vi "Maxi Gauge-Driver Core.vi"(0 "VISA-Ressource in":refnum<visa-resource-name>, 1 "Write/Read":bool, 5 "Node address":i8=-1 min=-1 max=31 step=1, 7 "Command":string, 11 "Fehler (Eingang)":errorcluster, 12 "Timeout [ms]":u32=600 min=1 max=20000 step=1, 13 "Retry (3)":i32=3 min=1 max=20000 step=1) -> (4 "VISA-Ressource out":refnum<visa-resource-name>, 8 "String Out":string, 15 "Fehler (Ausgang)":errorcluster)   [LabVIEW 2018, in "Maxi Gauge.lvlib"]
uses:
  Maxi Gauge.lvlib
panel:
  in  "ENQ [\\05]":string="\u0005"
  in  "NAK [\\15]":string="\u0015"
  in  "ACK [\\06]":string="\u0006"
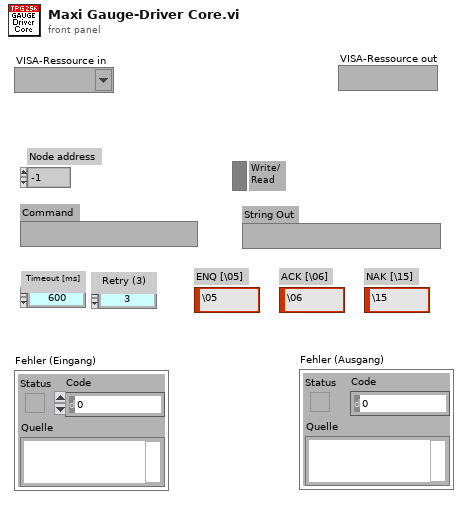
[diagram p1: front panel]
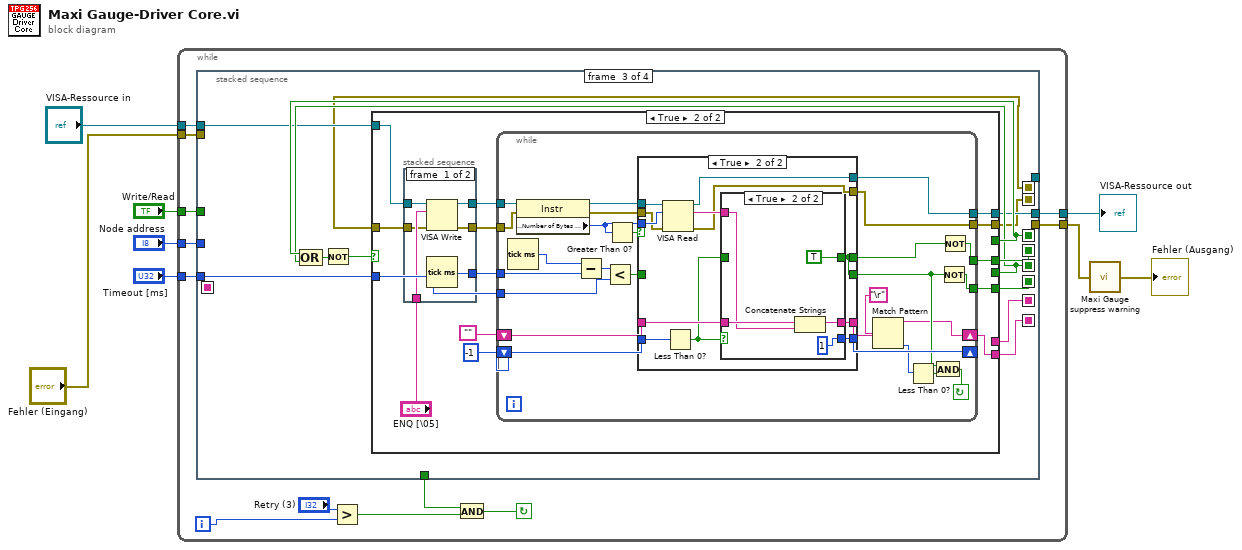
[diagram p0: block diagram]
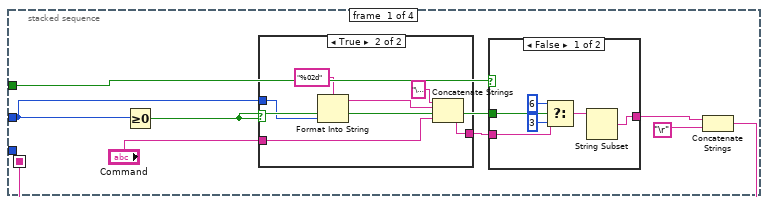
[diagram p2: hidden frame]
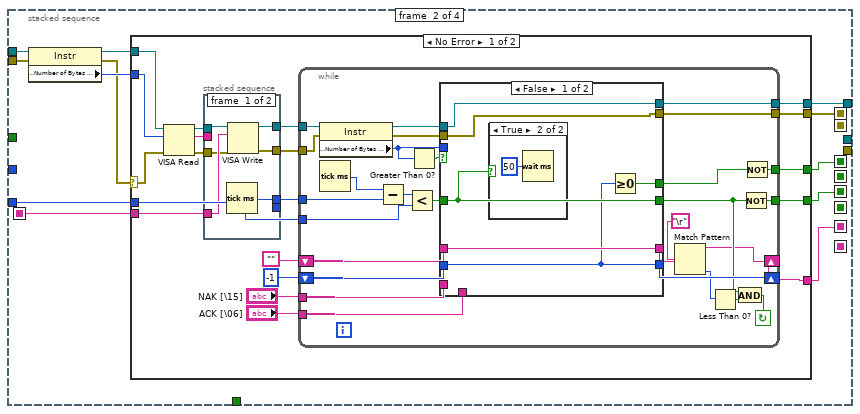
[diagram p5: hidden frame]
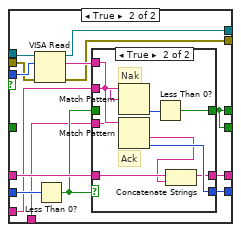
[diagram p7: hidden frame]
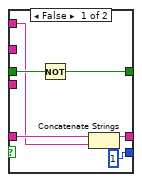
[diagram p8: hidden frame]
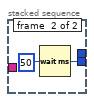
[diagram p9: hidden frame]
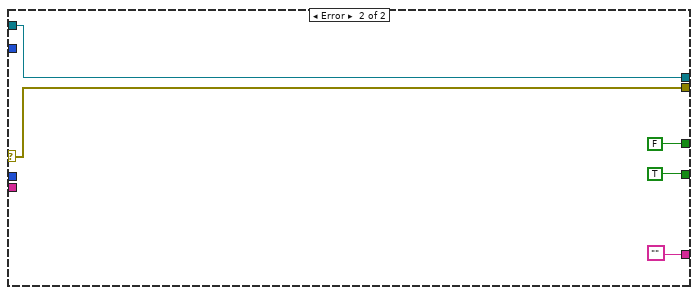
[diagram p10: hidden frame]
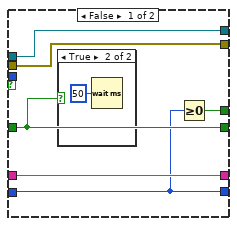
[diagram p12: hidden frame]
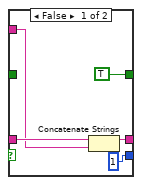
[diagram p14: hidden frame]
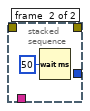
[diagram p15: hidden frame]
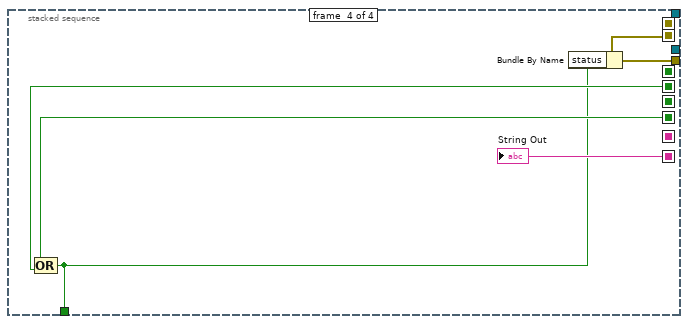
[diagram p16: hidden frame]
diagram:
  n1 = while {
    tunnel: "Node address" -> [w13]
    tunnel: "Write/Read" -> [w14]
    tunnel: "Timeout [ms]" -> [w20]
    tunnel: "VISA-Ressource in" -> [w12]
    tunnel: "Fehler (Eingang)" -> [w11]
    tunnel: [w10] -> w3
    tunnel: [w9] -> w2
    i -> [w18]
    stop <- w15 continue-if-true
    n2 = stacked-sequence {
      seq-local: [w28 _ _ _] -> [_ w52 _ _]
      seq-local: [_ w54 _ _] -> [_ _ w156 _]
      seq-local: [_ w50 _ _] -> [_ _ w158 _]
      seq-local: [_ w51 _ _] -> [_ _ w157 _]
      seq-local: [_ _ w163 _] -> [_ _ _ w249]
      seq-local: [_ _ w162 _] -> [_ _ _ w250]
      seq-local: [_ _ w161 _] -> [_ _ _ w251]
      seq-local: [_ w44 _ _] -> [_ _ w154 _]
      seq-local: [_ _ w152 _] -> [_ _ _ w248]
      tunnel: w20 -> [_ w53 w164 _]
      tunnel: [_ _ _ w247] -> w16
      tunnel: w14 -> [w25 _ _ _]
      tunnel: w13 -> [w27 _ _ _]
      tunnel: w12 -> [_ w49 w155 _]
      tunnel: w11 -> [_ w45 _ _]
      tunnel: [_ w43 _ _] -> _
      tunnel: [_ _ w153 _] -> w10
      tunnel: [_ _ _ w246] -> w9
      frame #0 {
        n3 = Greater Or Equal To 0?(x=w27) -> (x >= 0?=w22:bool)
        n4 = case shown="True" w22 {
          tunnel: w27 -> [_ w39]
          tunnel: [w36 w40] -> w24
          tunnel: "Command" -> [w36 w41]
          frame False {
          }
          frame True {
            n5 = Format Into String(format string="%02d", w39) -> (resulting string=w38:string)  [unwired: 2 in, 1 out]
            n6 = Concatenate Strings("\u001b", w38, w41) -> (w40:string)
          }
        }
        n7 = case shown="False" w25 {
          tunnel: w24 -> [w34 w35]
          tunnel: [w33 w35] -> w23
          tunnel: w22 -> [w30 _]
          frame False {
            n8 = Select(t=u8 6, s=w30, f=u8 3 ("t")) -> (s? t:f=w29:u8)
            n9 = String Subset(string=w34, length (rest)=w29) -> (substring=w33:string)  [unwired: 1 in]
          }
          frame True {
          }
        }
        n10 = Concatenate Strings(w23, "\r") -> (w28:string)
      }
      frame #1 {
        n11 = property class="Instr"(reference=w49, error in=w45) -> (reference out=w48:refnum<visa-resource-name>, error out=w46:errorcluster, "Serial Settings:Number of Bytes at Serial Port"=w47:u32)
        n12 = case shown="No Error" w46 {
          selector: w46 -> [w60 w148]
          tunnel: [w74 FALSE] -> w50
          tunnel: [w73 TRUE] -> w51
          tunnel: w52 -> [w69 _]
          tunnel: w53 -> [w68 _]
          tunnel: [w66 ""] -> w54
          tunnel: w48 -> [w64 w147]
          tunnel: w47 -> [w62 _]
          tunnel: [w56 w147] -> w43
          tunnel: [w55 w148] -> w44
          frame No Error {
            n13 = VISA Read(VISA resource name=w64, byte count=w62, error in (no error)=w60) -> (VISA resource name out=w63:refnum<visa-resource-name>, read buffer=w61:string, error out=w59:errorcluster)  [unwired: 1 out]
            n14 = stacked-sequence {
              tunnel: w69 -> [w142 _]
              tunnel: [w144 _] -> w67
              tunnel: [_ w145] -> _
              tunnel: w63 -> [w143 _]
              tunnel: w61 -> [_ _]
              tunnel: w59 -> [w141 _]
              tunnel: [w140 _] -> w58
              tunnel: [w139 _] -> w57
              frame #0 {
                n15 = Tick Count (ms)() -> (millisecond timer value=w144:u32)
                n16 = VISA Write(VISA resource name=w143, write buffer=w142, error in (no error)=w141) -> (VISA resource name out=w140:refnum<visa-resource-name>, error out=w139:errorcluster)  [unwired: 1 out]
              }
              frame #1 {
                n17 = Wait (ms)(milliseconds to wait=u32 50) -> (millisecond timer value=w145:u32)
              }
            }
            n18 = while {
              tunnel: "ACK [\\06]" -> [w87]
              tunnel: "NAK [\\15]" -> [w88]
              tunnel: [w89] -> w74
              tunnel: [w91] -> w73
              shift-left: -1 -> [w95]
              shift-right: [w94] -> _
              shift-left: "" -> [w96]
              shift-right: [w85] -> w66
              tunnel: w67 -> [w97]
              tunnel: w68 -> [w101]
              tunnel: w58 -> [w81]
              tunnel: w57 -> [w80]
              tunnel: [w77] -> w56
              tunnel: [w75] -> w55
              stop <- w93 continue-if-true
              n19 = property class="Instr"(reference=w81, error in=w80) -> (reference out=w79:refnum<visa-resource-name>, error out=w76:errorcluster, "Serial Settings:Number of Bytes at Serial Port"=w78:u32)
              n20 = Tick Count (ms)() -> (millisecond timer value=w98:u32)
              n21 = Subtract(x=w98, y=w97) -> (x-y=w102:u32)
              n22 = Less?(x=w102, y=w101) -> (x < y?=w99:bool)
              n23 = Greater Than 0?(x=w78) -> (x > 0?=w100:bool)
              n24 = case shown="False" w100 {
                tunnel: w78 -> [_ w114]
                tunnel: w99 -> [w107 _]
                tunnel: w96 -> [w108 w122]
                tunnel: w95 -> [w105 w123]
                tunnel: [w105 w121] -> w94
                tunnel: [w108 w120] -> w86
                tunnel: [w107 w116] -> w92
                tunnel: [w106 w116] -> w90
                tunnel: w88 -> [_ w118]
                tunnel: w87 -> [_ w117]
                tunnel: w79 -> [w104 w115]
                tunnel: [w104 w112] -> w77
                tunnel: w76 -> [w103 w111]
                tunnel: [w103 w110] -> w75
                frame False {
                  n25 = case shown="True" w107 {
                    frame False {
                    }
                    frame True {
                      n26 = Wait (ms)(milliseconds to wait=u32 50) -> ()  [unwired: 1 out]
                    }
                  }
                  n27 = Greater Or Equal To 0?(x=w105) -> (x >= 0?=w106:bool)
                }
                frame True {
                  n28 = VISA Read(VISA resource name=w115, byte count=w114, error in (no error)=w111) -> (VISA resource name out=w112:refnum<visa-resource-name>, read buffer=w113:string, error out=w110:errorcluster)  [unwired: 1 out]
                  n29 = Less Than 0?(x=w123) -> (x < 0?=w119:bool)
                  n30 = case shown="True" w119 {
                    tunnel: w113 -> [w124 w135]
                    tunnel: w122 -> [w129 w138]
                    tunnel: [1 w137] -> w121
                    tunnel: [w128 w136] -> w120
                    tunnel: [w125 w133] -> w116
                    tunnel: w119 -> [w126 _]
                    tunnel: w118 -> [_ w131]
                    tunnel: w117 -> [_ w130]
                    frame False {
                      n31 = Not(x=w126) -> (.not. x?=w125:bool)
                      n32 = Concatenate Strings(w129, w124) -> (w128:string)
                    }
                    frame True {
                      # "Ack"
                      # "Nak"
                      n33 = Match Pattern(string=w135, regular expression=w131) -> (offset past match=w134:i32)  [unwired: 1 in, 3 out]
                      n34 = Match Pattern(string=w135, regular expression=w130) -> (after substring=w132:string, offset past match=w137:i32)  [unwired: 1 in, 2 out]
                      n35 = Less Than 0?(x=w134) -> (x < 0?=w133:bool)
                      n36 = Concatenate Strings(w138, w132) -> (w136:string)
                    }
                  }
                }
              }
              n37 = Match Pattern(string=w86, regular expression="\r") -> (before substring=w85:string, offset past match=w82:i32)  [unwired: 1 in, 2 out]
              n38 = Less Than 0?(x=w82) -> (x < 0?=w83:bool)
              n39 = And(x=w92, y=w83) -> (x .and. y?=w93:bool)
              n40 = Not(x=w92) -> (.not. x?=w91:bool)
              n41 = Not(x=w90) -> (.not. x?=w89:bool)
            }
          }
          frame Error {
          }
        }
      }
      frame #2 {
        n42 = Compound Arithmetic op=OR(w158, w157) -> (w160:bool)
        n43 = Not(x=w160) -> (.not. x?=w159:bool)
        n44 = case shown="True" w159 {
          tunnel: w164 -> [_ w182]
          tunnel: [w169 w178] -> w163
          tunnel: [w168 w177] -> w162
          tunnel: [w167 w176] -> w161
          tunnel: w158 -> [w169 _]
          tunnel: w157 -> [w168 _]
          tunnel: w156 -> [w167 _]
          tunnel: w155 -> [w166 w175]
          tunnel: w154 -> [w165 w173]
          tunnel: [w166 w171] -> w153
          tunnel: [w165 w170] -> w152
          frame False {
          }
          frame True {
            n45 = stacked-sequence {
              tunnel: "ENQ [\\05]" -> [w242 _]
              tunnel: [w244 _] -> w181
              tunnel: w175 -> [w243 _]
              tunnel: [w241 _] -> w174
              tunnel: w173 -> [w240 _]
              tunnel: [w239 _] -> w172
              frame #0 {
                n46 = VISA Write(VISA resource name=w243, write buffer=w242, error in (no error)=w240) -> (VISA resource name out=w241:refnum<visa-resource-name>, error out=w239:errorcluster)  [unwired: 1 out]
                n47 = Tick Count (ms)() -> (millisecond timer value=w244:u32)
              }
              frame #1 {
                n48 = Wait (ms)(milliseconds to wait=u32 50) -> ()  [unwired: 1 out]
              }
            }
            n49 = while {
              tunnel: [w191] -> w177
              tunnel: [w192] -> w178
              shift-left: -1 -> [w202]
              shift-right: [w201] -> _
              shift-left: "" -> [w203]
              shift-right: [w196] -> w176
              tunnel: w181 -> [w204]
              tunnel: w182 -> [w208]
              tunnel: w174 -> [w188]
              tunnel: w172 -> [w189]
              tunnel: [w185] -> w171
              tunnel: [w184] -> w170
              stop <- w200 continue-if-true
              n50 = Tick Count (ms)() -> (millisecond timer value=w205:u32)
              n51 = property class="Instr"(reference=w188, error in=w189) -> (reference out=w187:refnum<visa-resource-name>, error out=w186:errorcluster, "Serial Settings:Number of Bytes at Serial Port"=w190:u32)
              n52 = Subtract(x=w205, y=w204) -> (x-y=w209:u32)
              n53 = Less?(x=w209, y=w208) -> (x < y?=w206:bool)
              n54 = Greater Than 0?(x=w190) -> (x > 0?=w207:bool)
              n55 = case shown="True" w207 {
                tunnel: w190 -> [_ w221]
                tunnel: w206 -> [w214 _]
                tunnel: w203 -> [w215 w227]
                tunnel: w202 -> [w212 w228]
                tunnel: [w212 w226] -> w201
                tunnel: [w215 w225] -> w197
                tunnel: [w214 w223] -> w199
                tunnel: [w213 w223] -> w198
                tunnel: w187 -> [w211 w222]
                tunnel: w186 -> [w210 w220]
                tunnel: [w211 w218] -> w185
                tunnel: [w210 w217] -> w184
                frame False {
                  n56 = case shown="True" w214 {
                    frame False {
                    }
                    frame True {
                      n57 = Wait (ms)(milliseconds to wait=u32 50) -> ()  [unwired: 1 out]
                    }
                  }
                  n58 = Greater Or Equal To 0?(x=w212) -> (x >= 0?=w213:bool)
                }
                frame True {
                  n59 = VISA Read(VISA resource name=w222, byte count=w221, error in (no error)=w220) -> (VISA resource name out=w218:refnum<visa-resource-name>, read buffer=w219:string, error out=w217:errorcluster)  [unwired: 1 out]
                  n60 = Less Than 0?(x=w228) -> (x < 0?=w224:bool)
                  n61 = case shown="True" w224 {
                    tunnel: w219 -> [w230 w236]
                    tunnel: w227 -> [w233 w238]
                    tunnel: [1 1] -> w226
                    tunnel: [w232 w237] -> w225
                    tunnel: [TRUE TRUE] -> w223
                    tunnel: w224 -> [_ _]
                    frame False {
                      n62 = Concatenate Strings(w233, w230) -> (w232:string)
                    }
                    frame True {
                      n63 = Concatenate Strings(w238, w236) -> (w237:string)
                    }
                  }
                }
              }
              n64 = Match Pattern(string=w197, regular expression="\r") -> (before substring=w196:string, offset past match=w193:i32)  [unwired: 1 in, 2 out]
              n65 = Less Than 0?(x=w193) -> (x < 0?=w194:bool)
              n66 = And(x=w199, y=w194) -> (x .and. y?=w200:bool)
              n67 = Not(x=w199) -> (.not. x?=w191:bool)
              n68 = Not(x=w198) -> (.not. x?=w192:bool)
            }
          }
        }
      }
      frame #3 {
        n69 = Compound Arithmetic op=OR(w250, w249) -> (w247:bool)
        n70 = Bundle By Name(cluster=w248, "status"=w247) -> (w246:errorcluster)
        "String Out" <- w251
      }
    }
    n71 = Greater?(x="Retry (3)", y=w18) -> (0:w17:bool)
    n72 = And(x=w16, y=w17) -> (x .and. y?=w15:bool)
  }
  "VISA-Ressource out" <- w3
  n73 = call "Maxi Gauge suppress warning.vi"("error in"=w2) -> ("error out"=→"Fehler (Ausgang)":errorcluster)
